vi "Turn Crank.vi"(0 "reference in":refnum<class "Gum Machine.lvclass">, 5 "error in (no error)":errorcluster) -> (14 "reference out":refnum<class "Gum Machine.lvclass">, 19 "error out":errorcluster)   [LabVIEW 2013, in "Gum Machine.lvclass"]
uses:
  Gum Machine.lvclass
  State_class/State.lvclass
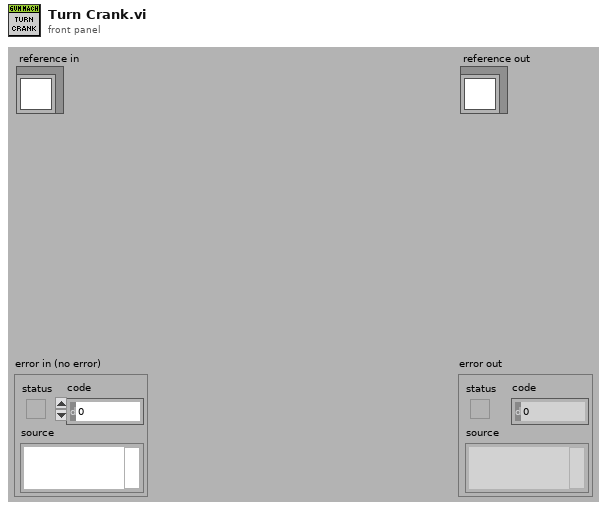
[diagram p1: front panel]
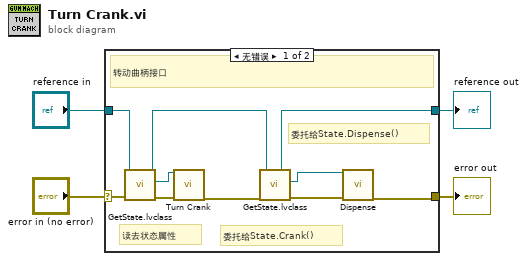
[diagram p0: block diagram]
diagram:
  n1 = case shown="无错误" "error in (no error)" {
    selector: "error in (no error)" -> [w13 w16]
    tunnel: [w10 w16] -> w3
    tunnel: [w7 w15] -> w1
    tunnel: "reference in" -> [w14 w15]
    frame No Error {
      # "委托给State.Dispense()"
      # "委托给State.Crank()"
      # "读去状态属性"
      # "转动曲柄接口"
      n2 = call-dynamic "GetState.lvclass.vi"("error in (no error)"=w13, "reference in"=w14) -> ("error out"=w11:errorcluster, "State.lvclass"=w12:refnum<class "State.lvclass">, "reference out"=w8:refnum<class "Gum Machine.lvclass">)  [unwired: 7 in]
      n3 = call-dynamic "Turn Crank.vi"("reference in"=w12, "error in (no error)"=w11) -> ("error out"=w9:errorcluster)  [unwired: 16 in, 1 out]
      n4 = call-dynamic "GetState.lvclass.vi"("error in (no error)"=w9, "reference in"=w8) -> ("error out"=w6:errorcluster, "State.lvclass"=w5:refnum<class "State.lvclass">, "reference out"=w7:refnum<class "Gum Machine.lvclass">)  [unwired: 7 in]
      n5 = call-dynamic "Dispense.vi"("reference in"=w5, "error in (no error)"=w6) -> ("error out"=w10:errorcluster)  [unwired: 16 in, 1 out]
    }
    frame Error {
    }
  }
  "error out" <- w3
  "reference out" <- w1
